vi "Module Loop.vi"(8 "error in (no error)":errorcluster, 11 "HTTP Command Bridge in":refnum<class "HTTP Command Bridge.lvclass">) -> (0 "error out":errorcluster, 3 "HTTP Command Bridge out":refnum<class "HTTP Command Bridge.lvclass">)   [LabVIEW 2020, in "Volatus.lvlib" / "HTTP Command Bridge.lvclass"]
uses:
  HTTP Command Bridge.lvclass
  C:/dev/lv20CE/relink/lv-volatus/Volatus/Module/Module.lvclass
  Module/Module.lvclass
  Http Chan Cmd.ctl
  Http Cmd Type.ctl
  Module/Module.lvclass/Module.ctl
  <vilib>/Utility/error.llb/Error Cluster From Error Code.vi
  lv-promises/Promises/Promise/Promise.lvclass
  HTTP Command Bridge.lvclass/HTTP Command Bridge.ctl
  MessageQ/MessageQ.lvclass
  Volatus.lvlib
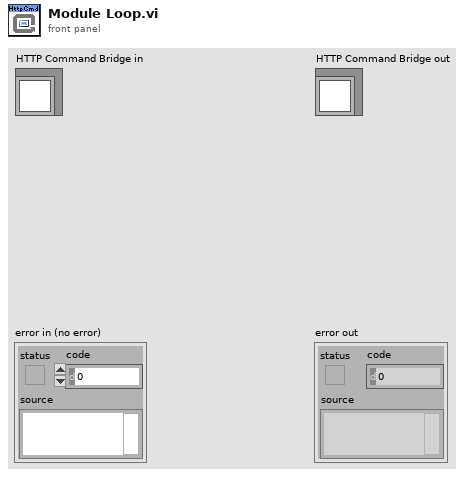
[diagram p1: front panel]
types:
  T1 = enum32{"Invalid", "Standard", "Closed", "Hidden", "Minimized", "Maximized"}
  T2 = typedef "Volatus.lvlib/Http Chan Cmd.ctl" = cluster{"Type":T3, "Channel":string, "Value":dbl}
  T3 = typedef "Volatus.lvlib/Http Cmd Type.ctl" = enum16{"Digital", "Numeric"}
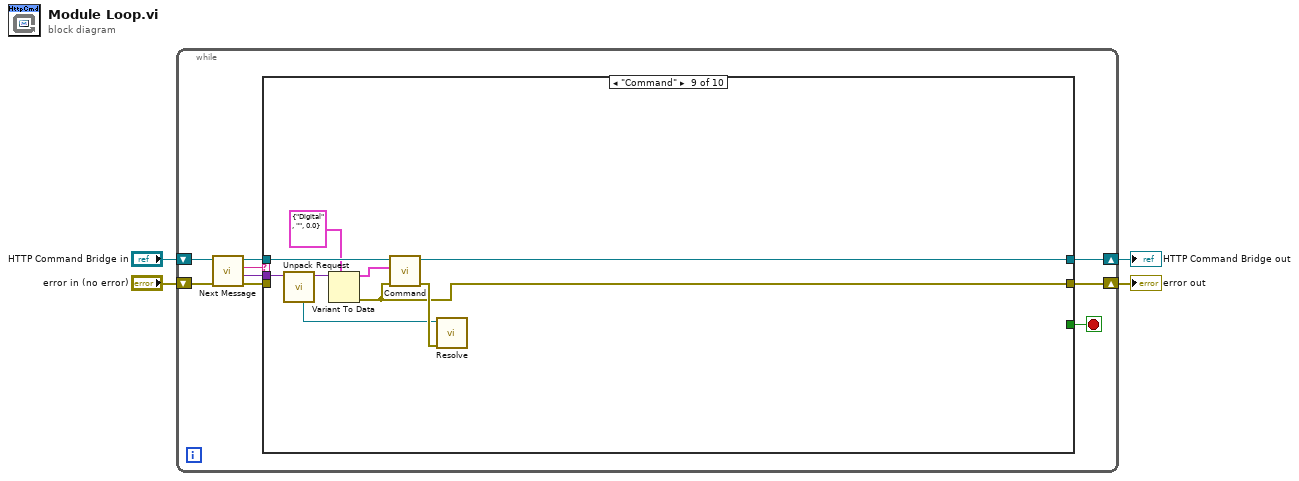
[diagram p0: block diagram]
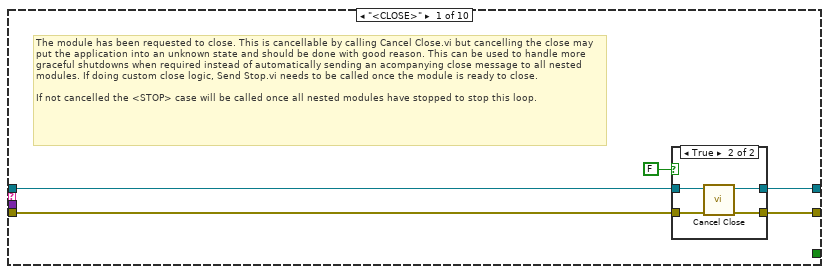
[diagram p2: hidden frame]
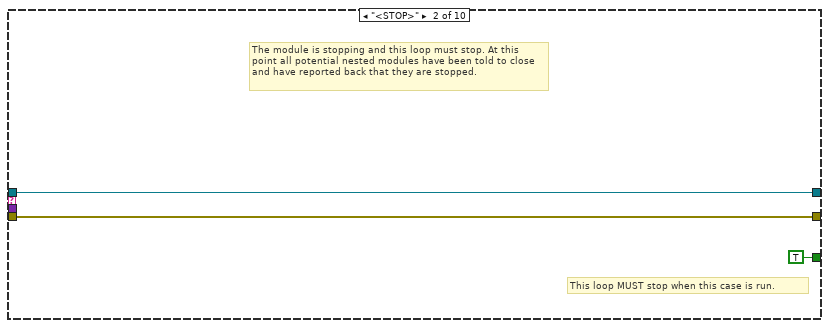
[diagram p4: hidden frame]
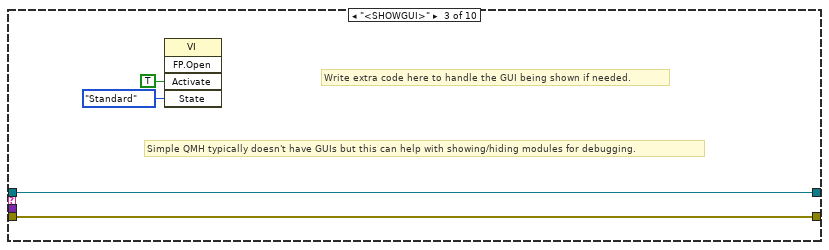
[diagram p5: hidden frame]
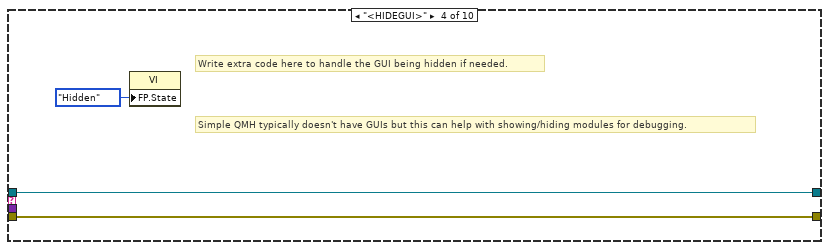
[diagram p6: hidden frame]
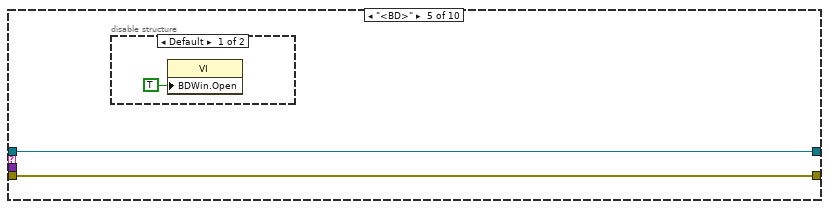
[diagram p7: hidden frame]
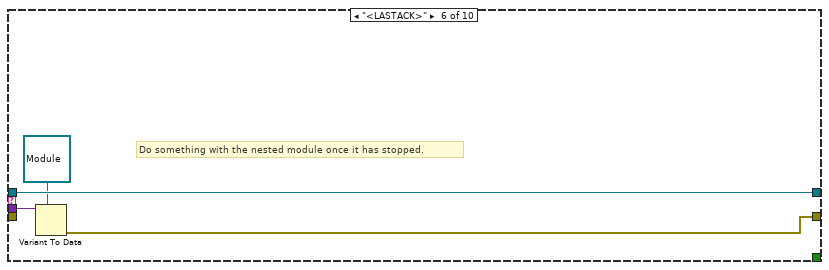
[diagram p9: hidden frame]
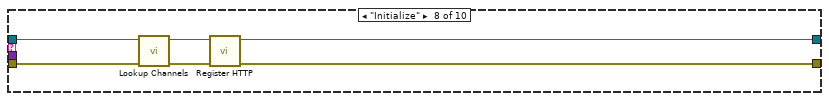
[diagram p11: hidden frame]
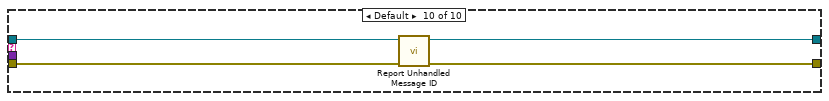
[diagram p12: hidden frame]
diagram:
  n1 = while {
    shift-right: [w8] -> w2
    shift-left: "HTTP Command Bridge in" -> [w13]
    shift-right: [w7] -> w1
    shift-left: "error in (no error)" -> [w12]
    stop <- w6 stop-if-true
    n2 = call "Next Message.vi"("error in (no error)"=w12, "Module in"=w13) -> ("error out"=w11:errorcluster, "Data"=w5:variant, "ID"=w10:string, "Module out"=w9:refnum<class "HTTP Command Bridge.lvclass">)  [unwired: 6 in]
    n3 = case shown="\"Command\"" w10 {
      tunnel: w11 -> [w18 w26 w30 w33 w35 _ w42 w49 _ w62]
      tunnel: w9 -> [w16 w27 w31 w34 w36 w41 w43 w47 w57 w60]
      tunnel: [w15 w27 w31 w34 w36 w41 w43 w44 w52 w59] -> w8
      tunnel: [w17 w26 w30 w33 w35 w38 w42 w46 w50 w61] -> w7
      tunnel: [_ TRUE _ _ _ _ _ _ _ _] -> w6
      tunnel: w5 -> [_ _ _ _ _ w40 _ _ w56 _]
      frame "<CLOSE>" {
        # "The module has been requested to close. This is cancellable by calling Cancel Close.vi but cancelling the close may put the application into an unknown state and should be done with good reason. This can be used to handle more graceful shutdowns when required instead of automatically sending an acompanying close message to all nested modules. If doing custom close logic, Send Stop.vi needs to be called once the module is ready to close.\n\nIf not cancelled the <STOP> case will be called once all nested modules have stopped to stop this loop."
        n4 = case shown="True" FALSE {
          tunnel: w18 -> [w19 w24]
          tunnel: [w19 w23] -> w17
          tunnel: w16 -> [w20 w22]
          tunnel: [w20 w21] -> w15
          frame False {
          }
          frame True {
            n5 = call "Cancel Close.vi"("error in (no error)"=w24, "Module in"=w22) -> ("error out"=w23:errorcluster, "Module out"=w21:refnum<class "HTTP Command Bridge.lvclass">)  [unwired: 8 in]
          }
        }
      }
      frame "<STOP>" {
        # "This loop MUST stop when this case is run."
        # "The module is stopping and this loop must stop. At this point all potential nested modules have been told to close and have reported back that they are stopped."
      }
      frame "<SHOWGUI>" {
        # "Simple QMH typically doesn't have GUIs but this can help with showing/hiding modules for debugging."
        # "Write extra code here to handle the GUI being shown if needed."
        n6 = invoke class="VI" method="FP.Open"("Activate"=TRUE ("Activate?"), "State"=T1."Standard") -> ()  [unwired: 3 in, 5 out]
      }
      frame "<HIDEGUI>" {
        # "Simple QMH typically doesn't have GUIs but this can help with showing/hiding modules for debugging."
        # "Write extra code here to handle the GUI being hidden if needed."
        n7 = property class="VI"("FP.State"=T1."Hidden" ("Front Panel Window:State")) -> ()  [unwired: 2 in, 2 out]
      }
      frame "<BD>" {
        n8 = disable-structure shown="Default" {
          frame condition #0 (active) {
            n9 = property class="VI"("BDWin.Open"=TRUE ("Block Diagram Window:Open")) -> ()  [unwired: 2 in, 2 out]
          }
          frame condition #1 {
          }
        }
      }
      frame "<LASTACK>" {
        # "Do something with the nested module once it has stopped."
        n10 = Variant To Data(type=refnum<class "Module.lvclass"> refnum ("Volatus:Module"), Variant=w40) -> (error out=w38:errorcluster)  [unwired: 1 in, 1 out]
      }
      frame "<TIMEOUT>" {
        # "No message for this module was received in time"
      }
      frame "Initialize" {
        n11 = call "Lookup Channels.vi"("error in (no error)"=w49, "HTTP Command Bridge in"=w47) -> ("error out"=w48:errorcluster, "HTTP Command Bridge out"=w45:refnum<class "HTTP Command Bridge.lvclass">)  [unwired: 8 in]
        n12 = call "Register HTTP.vi"("error in (no error)"=w48, "HTTP Command Bridge in"=w45) -> ("error out"=w46:errorcluster, "HTTP Command Bridge out"=w44:refnum<class "HTTP Command Bridge.lvclass">)  [unwired: 8 in]
      }
      frame "Command" {
        n13 = call "Unpack Request.vi"("Request Data"=w56) -> ("Data"=w55:variant, "Promise"=w53:refnum<class "Promise.lvclass">)  [unwired: 8 in, 1 out]
        n14 = Variant To Data(type=T2 {"Type"=enum."Digital", "Channel"="", "Value"=0.0} ("Http Chan Cmd"), Variant=w55) -> (data=w51:T2, error out=w50:errorcluster)  [unwired: 1 in]
        n15 = call "Command.vi"("error in (no error)"=w50, "Http Chan Cmd"=w51, "HTTP Command Bridge in"=w57) -> ("error out"=w58:errorcluster, "HTTP Command Bridge out"=w52:refnum<class "HTTP Command Bridge.lvclass">)  [unwired: 7 in]
        n16 = call "Resolve.vi"("error in (no error)"=w58, "Promise in"=w53) -> ()  [unwired: 8 in, 2 out]
      }
      frame Default {
        n17 = call "Report Unhandled Message ID.vi"("error in (no error)"=w62, "Module in"=w60) -> ("error out"=w61:errorcluster, "Module out"=w59:refnum<class "HTTP Command Bridge.lvclass">)  [unwired: 8 in]
      }
    }
  }
  "error out" <- w1
  "HTTP Command Bridge out" <- w2
